vi "Alignment Apply Offset SLM.vi"(11 "current offset":dbl) -> ()   [LabVIEW 2014]
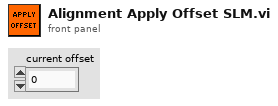
[diagram p1: front panel]
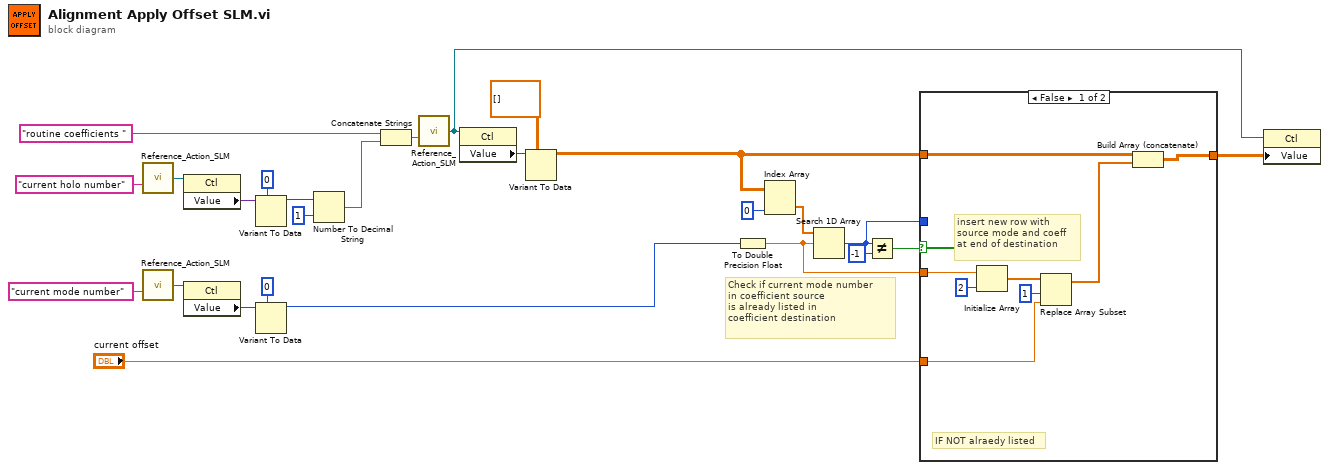
[diagram p0: block diagram]
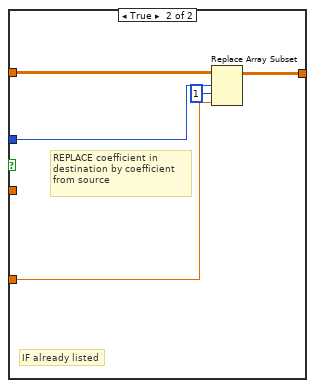
[diagram p2: hidden frame]
diagram:
  # "Check if current mode number \nin coefficient source\nis already listed in \ncoefficient destination"
  n1 = call "Reference_Action_SLM.vi"("Control Name"="current holo number") -> ("Ref OUT"=w23:refnum<vi>)  [unwired: 12 in, 2 out]
  n2 = call "Reference_Action_SLM.vi"("Control Name"="current mode number") -> ("Ref OUT"=w17:refnum<vi>)  [unwired: 12 in, 2 out]
  n3 = property class="Ctl"(reference=w23) -> ("Value"=w22:variant)  [unwired: 1 in, 2 out]
  n4 = property class="Ctl"(reference=w17) -> ("Value"=w16:variant)  [unwired: 1 in, 2 out]
  n5 = Variant To Data(type=0 ("disabled index (col)"), Variant=w22) -> (data=w20:i32)  [unwired: 1 in, 1 out]
  n6 = Variant To Data(type=0 ("disabled index (col)"), Variant=w16) -> (data=w3:i32)  [unwired: 1 in, 1 out]
  n7 = Number To Decimal String(number=w20, width (-)=i16 1) -> (decimal integer string=w13:string)
  n8 = Concatenate Strings("routine coefficients " ("Control Name"), w13) -> (w14:string)
  n9 = call "Reference_Action_SLM.vi"("Control Name"=w14) -> ("Ref OUT"=w2:refnum<vi>)  [unwired: 12 in, 2 out]
  n10 = property class="Ctl"(reference=w2) -> ("Value"=w26:variant)  [unwired: 1 in, 2 out]
  n11 = Variant To Data(type=dbl[][] [] ("collapsed mode array"), Variant=w26) -> (data=w5:dbl[][])  [unwired: 1 in, 1 out]
  n12 = To Double Precision Float(number=w3) -> (double precision float=w6:dbl)
  n13 = Index Array(array=w5, index (col)=0 ("disabled index (col)")) -> (element=w10:dbl[])  [unwired: 1 in]
  n14 = Search 1D Array(1D array=w10, element=w6) -> (index of element=w7:i32)  [unwired: 1 in]
  n15 = Not Equal?(x=w7, y=-1) -> (x != y?=w8:bool)
  n16 = case shown="False" w8 {
    tunnel: w7 -> [_ w38]
    tunnel: w5 -> [w29 w35]
    tunnel: "current offset" -> [w30 w36]
    tunnel: [w28 w37] -> w1
    tunnel: w6 -> [w33 _]
    frame False {
      # "insert new row with \nsource mode and coeff\nat end of destination"
      # "IF NOT alraedy listed"
      n17 = Initialize Array(w33, 2 ("dimension size")) -> (w32:dbl[])
      n18 = Replace Array Subset(array=w32, new element=w30, index=1) -> (w27:dbl[])
      n19 = Build Array (concatenate)(w29, w27) -> (w28:dbl[][])
    }
    frame True {
      # "REPLACE coefficient in \ndestination by coefficient \nfrom source"
      # "IF already listed"
      n20 = Replace Array Subset(array=w35, new element=w36, index (row)=w38, index (col)=1 ("disabled index (col)")) -> (w37:dbl[][])
    }
  }
  n21 = property class="Ctl"(reference=w2, "Value"=w1) -> ()  [unwired: 1 in, 2 out]
